vi "Launch Update from Git.vi"(8 "error in (no error)":errorcluster, 9 "Branch name":string, 10 "Update GIT":bool=TRUE, 11 "Guardian in":refnum<class "Guardian.lvclass">) -> (0 "error out":errorcluster, 3 "Guardian out":refnum<class "Guardian.lvclass">)   [LabVIEW 2026, in "TALOS.lvlib" / "Guardian.lvlib" / "Guardian.lvclass"]
uses:
  Guardian.lvclass
  Ancestor/Ancestor/Ancestor.lvclass/Ancestor.ctl
  Support VIs/Generate Error.vi
  FGV/Error Memory/Get Error Description.vi
  Support VIs/Get PC name.vi
  Ancestor/Ancestor/Read ID.vi
  Support VIs/Get Class Name.vi
  <vilib>/Utility/error.llb/Clear Errors.vi
  FGV/Error Memory/Error Memory Core.vi
  <vilib>/AdvancedString/Delimited String to 1D String Array.vi
  <vilib>/AdvancedString/Delimited String to 1D String Array (string).vi
  Support VIs/Circus Root Path.vi
  FGV/Error Memory/Error Crt Lvl checker.vi
  FGV/Error Memory/Error Memory Core.vi/40c8088d-b597-4017-91af-faa98e00292e.vi
  FGV/Error Memory/Error Memory Core.vi/d4a3ab98-063c-4e44-b43d-fbdcfe6c2be2.vi
  Update from GIT.vi
  Support VIs/Global Memory.vi
  <vilib>/Utility/LVClass/Get LV Class Name.vi
  Support VIs/Is in Packed Library.vi
  Support VIs/TALOS Root path.vi
  Support VIs/Read CSV worksheet.vi
  Support VIs/Global Constants.vi
  <vilib>/Utility/error.llb/General Error Handler.vi
  Support VIs/Error Log.vi
  Ancestor/Ancestor/Ancestor.lvclass
  <vilib>/Comparison/Equal/Equal Functor/Equal Functor.lvclass
  TALOS.lvlib
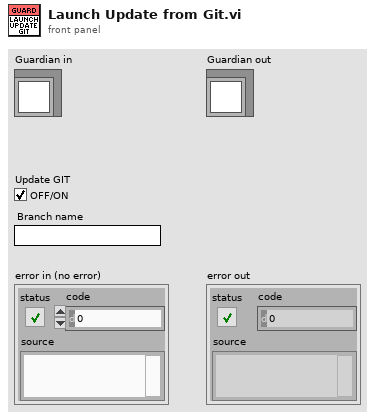
[diagram p1: front panel]
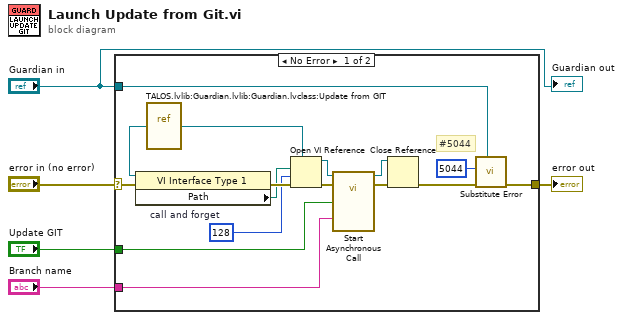
[diagram p0: block diagram]
diagram:
  n1 = case shown="No Error" "error in (no error)" {
    selector: "error in (no error)" -> [w14 w21]
    tunnel: [w9 w21] -> w5
    tunnel: "Guardian in" -> [w8 _]
    tunnel: "Branch name" -> [w7 _]
    tunnel: "Update GIT" -> [w6 _]
    frame No Error {
      w13 = 128  # call and forget
      # "#5044"
      n2 = vi-ref "TALOS.lvlib:Guardian.lvlib:Guardian.lvclass:Update from GIT.vi"() -> (w17:refnum<vi>)
      n3 = property class="VI Interface Type 1"(reference=w17, error in=w14) -> (error out=w15:errorcluster, "Path"=w12:path)  [unwired: 1 out]
      n4 = Open VI Reference(type specifier VI Refnum (for type only)=w17, vi path=w12, options=w13, error in (no error)=w15) -> (vi reference=w18:refnum<vi>, error out=w16:errorcluster)  [unwired: 2 in]
      n5 = call-by-ref "Start Asynchronous Call"(reference=w18, error in=w16, "Branch name"=w7, "Update GIT"=w6) -> (reference out=w19:refnum<vi>, error out=w20:errorcluster)  [unwired: 1 in]
      n6 = Close Reference(reference=w19, error in (no error)=w20) -> (error out=w10:errorcluster)
      n7 = call "Substitute Error.vi"("LabVIEW Object"=w8, "error in (no error)"=w10, "Error Code"=5044) -> ("error out"=w9:errorcluster)  [unwired: 8 in]
    }
    frame Error {
    }
  }
  "error out" <- w5
  "Guardian out" <- "Guardian in"
